vi "SetParam.vi"(8 "error in (no error)":errorcluster caption="entrée d'erreur (pas d'erreur)", 10 "make_hastie_10_2":T1={"n_samples"=12000, "random_state"=-1, "Returns"="X"} {"random_state" min=-1; "n_samples" min=1}, 11 "Hastie_10_2.lvclass":refnum<class "Hastie_10_2.lvclass">) -> (0 "error out":errorcluster caption="sortie d'erreur", 3 "Hastie_10_2.lvclass":refnum<class "Hastie_10_2.lvclass">)   [LabVIEW 2020, in "Hastie_10_2.lvclass"]
doc: "Set Parameters"
uses:
  Hastie_10_2.lvclass
  Hastie_10_2.lvclass/Hastie_10_2.ctl
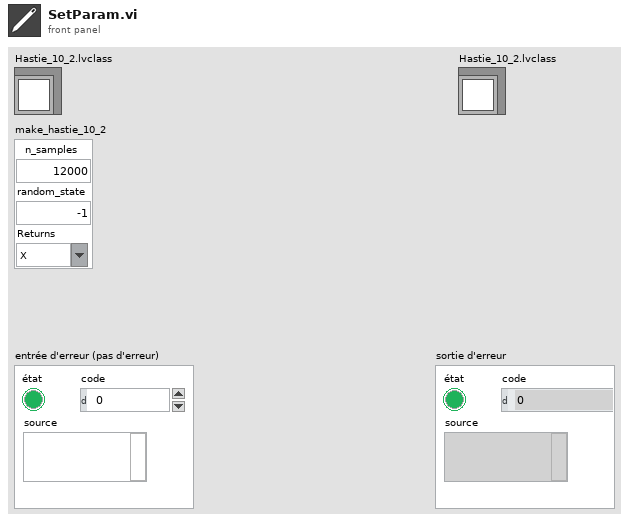
[diagram p1: front panel]
types:
  T1 = cluster{"n_samples":u32, "random_state":i32, "Returns":string}
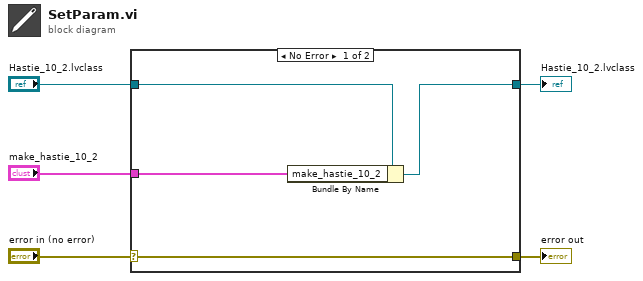
[diagram p0: block diagram]
diagram:
  n1 = case shown="No Error" "error in (no error)" {
    selector: "error in (no error)" -> [w9 w10]
    tunnel: [w9 w10] -> w4
    tunnel: [w7 w11] -> w2
    tunnel: "Hastie_10_2.lvclass" -> [w8 w11]
    tunnel: "make_hastie_10_2" -> [w6 _]
    frame No Error {
      n2 = Bundle By Name(cluster=w8, "make_hastie_10_2"=w6) -> (w7:refnum<class "Hastie_10_2.lvclass">)
    }
    frame Error {
    }
  }
  "error out" <- w4
  "Hastie_10_2.lvclass" <- w2
